vi "VoltageRatioInputSetBridgeGain.vi"(0 "error in (no error)":errorcluster, 2 "Bridge Gain":u32(ring)=8 items=["BRIDGE_GAIN_1"=1, "BRIDGE_GAIN_2"=2, "BRIDGE_GAIN_4"=3, "BRIDGE_GAIN_8"=4, "BRIDGE_GAIN_16"=5, "BRIDGE_GAIN_32"=6, "BRIDGE_GAIN_64"=7, "BRIDGE_GAIN_128"=8], 3 "Device In":u64) -> (7 "error out":errorcluster, 10 "Device Out":u64)   [LabVIEW 2020, in "Phidget Voltage Ratio Input.lvlib"]
doc: "${BridgeGain:Header}"
uses:
  <instrlib>/Phidgets/Phidget Voltage Ratio Input/Phidget Voltage Ratio Input.lvlib
  <instrlib>/Phidgets/Phidget Common/Phidget Common.lvlib
  phidget22.dll
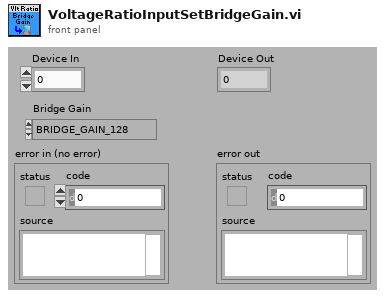
[diagram p1: front panel]
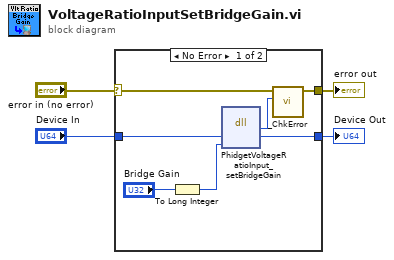
[diagram p0: block diagram]
diagram:
  n1 = case shown="No Error" "error in (no error)" {
    selector: "error in (no error)" -> [w9 w13]
    tunnel: [w8 w13] -> w3
    tunnel: "Device In" -> [w11 w12]
    tunnel: [w10 w12] -> w1
    frame No Error {
      n2 = To Long Integer(number="Bridge Gain") -> (32bit integer=w6:i32)
      n3 = dll-call lib="phidget22.*" fn="PhidgetVoltageRatioInput_setBridgeGain"("phid"=w11, "interval"=w6) -> ("return type"=w7:i32, "phid"=w10:u64)  [unwired: 4 in, 2 out]
      n4 = call <instrlib>:"_ChkError.vi"("Return Code"=w7, "error in (no error)"=w9) -> ("error out"=w8:errorcluster)  [unwired: 9 in]
    }
    frame Error {
    }
  }
  "error out" <- w3
  "Device Out" <- w1
